vi "General Error Handler CORE.vi"(0 "[error code] (0)":i32 format="%0.0f", 1 "[user-defined codes]":i32[](array[numeric]), 2 "[user-defined descriptions]":string[](array[string]), 5 "[error source] (\" \")":string, 7 "String to Format (not a refnum)":refnum<vi>, 9 "type of dialog (OK msg:1)":T2=enum."OK message", 11 "error in (no error)":errorcluster, 12 "[exception action] (none:0)":i32(ring) items=["no exception", "cancel error on match", "set error on match"], 13 "[exception code]":i32 format="%0.0f", 14 "[exception source]":string) -> (3 "stop event propagated":bool, 4 "error?":bool, 6 "code out":i32 format="%0.0f", 8 "source out":string, 10 "message":string=" INSTRUCTIONS:\r\rNormal Use:  When using subVIs that incorporate the error in/error out (or error I/O) structure, place this handler where you want to inform the user of an error, typically at the end of the I/O data path, as the last action of the program.  If the error in error? is ERROR, the handler creates a message describing the error and its source.  If the type of dialog = 1 (default), the message is displayed to the user, who can only acknowledge it.  If the type = 2, the user can acknowledge the message or abort execution; aborting a program with active I/O is not recommended.  If the type = 0, no message is displayed; this is used to process the error programmatically, and the error out cluster elements are wired to individual terminals for that reason.  \r\rOther Use:\n\r\nlocal testing.  To test the error code of a subVI or function that does not have the error I/O structure, you can wire its error code and a source string to the local error code and error source inputs.  If error in error? indicates no error and error code is not equal to 0, the local code and source are substituted for the error in values, and error? is set TRUE (ERROR).", 15 "error out":errorcluster)   [LabVIEW 2011]
doc: "Indicates whether an error occurred. If an error occurred, this VI returns a description of the error and optionally displays a dialog box."
uses:
  DialogTypeEnum.ctl
  whitespace.ctl
panel:
  in  "prompts":T1={"Error %d occurred at %s"="Error %d occurred at %s", "Warning %d occurred at %s"="Warning %d occurred at %s", "Possible reasons: %s"="<b>Possible reason(s):</b>\\n%s", "Error not listed"="This error code is undefined. No one has provided a description for this code, or you might have wired a number that is not an error code to the error code input.", "GetCommError x%lx"="Windows GetCommError:  The hex value of this code is <B>x%04lx</B>.\n\nInterpret it bit-wise as follows:\n<B>x4000</B>: serial port VI error\n<B>x0001</B>: receiving queue overflowed or character was received after end-of-file character\n<B>x0002</B>: character was lost by overwrite\n<B>x0004</B>: parity error\n<B>x0008</B>: framing error\n<B>x0010</B>: break condition\n<B>x0020</B>: CTS timeout\n<B>x0040</B>: DSR timeout\n<B>x0080</B>: RLSD timeout\n<B>x0100</B>: transmission queue was full when new character arrived\n<B>x0200</B>: parallel device timeout\n<B>x0400</B>: parallel device I/O error\n<B>x0800</B>: parallel device not selected\n<B>x1000</B>: parallel device out of paper\n<B>x8000</B>: requested mode is  not supported or the idComDev parameter is invalid.", "Continue"="Continue", "Stop"="Stop", "an unidentified location"="an unidentified location", "No Error"="No Error", "Help"="Why not found?"}
  # "reinitialize to default to display instructions"
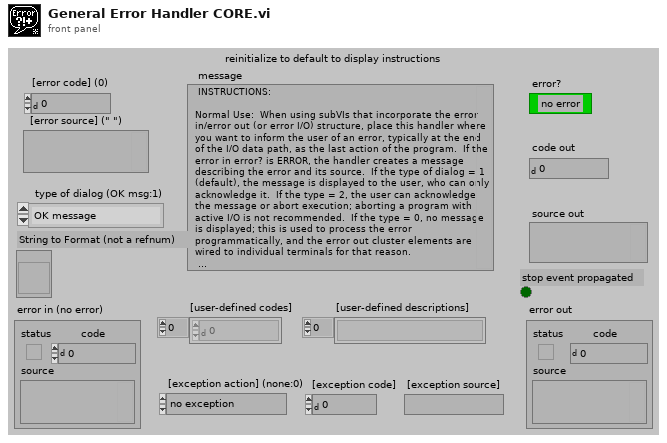
[diagram p1: front panel]
types:
  T1 = cluster{"Error %d occurred at %s":string, "Warning %d occurred at %s":string, "Possible reasons: %s":string, "Error not listed":string, "GetCommError x%lx":string, "Continue":string, "Stop":string, "an unidentified location":string, "No Error":string, "Help":string}
  T2 = typedef "DialogTypeEnum.ctl" = enum16{"no dialog", "OK message", "continue or stop message", "auto error handling dialog", "OK message + warnings", "continue/stop + warnings"}
  T3 = typedef "TagReturnType.ctl" = enum16{"No Tag", "<err>", "<append>"}
  T4 = typedef "whitespace.ctl" = u16
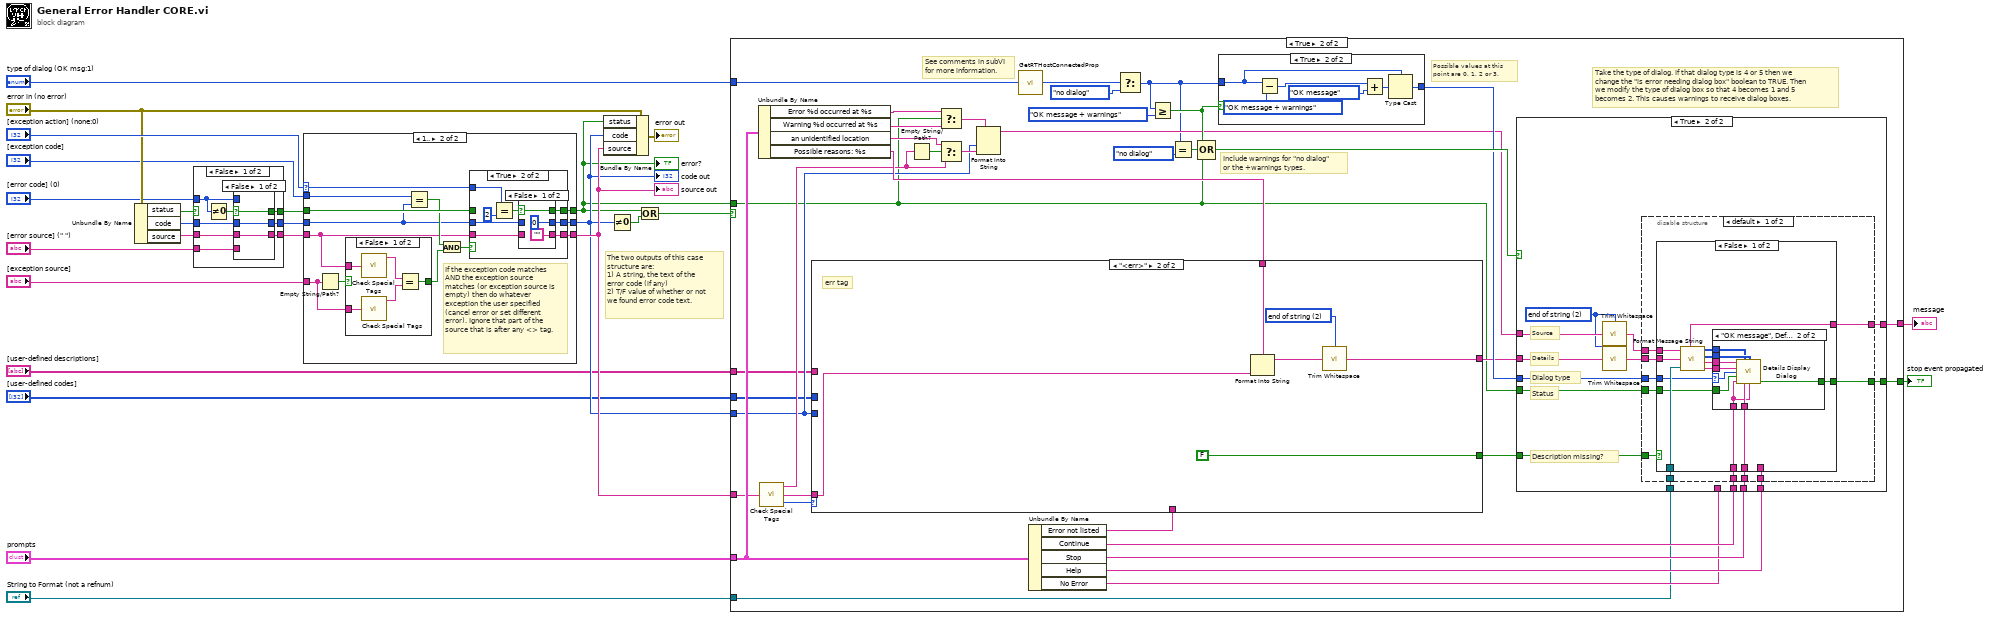
[diagram p0: block diagram]
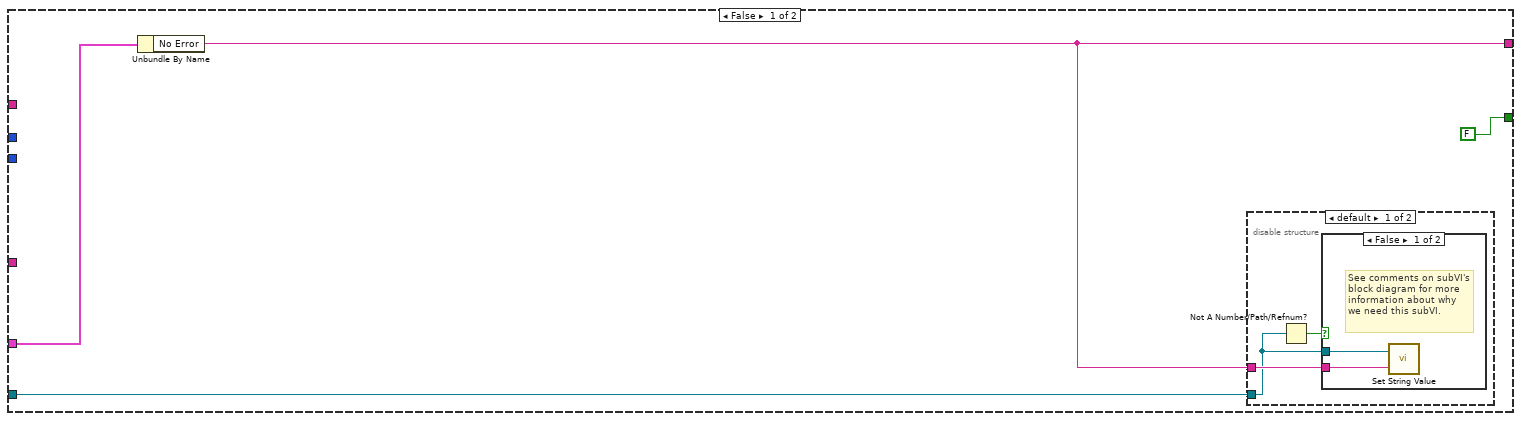
[diagram p8: hidden frame]
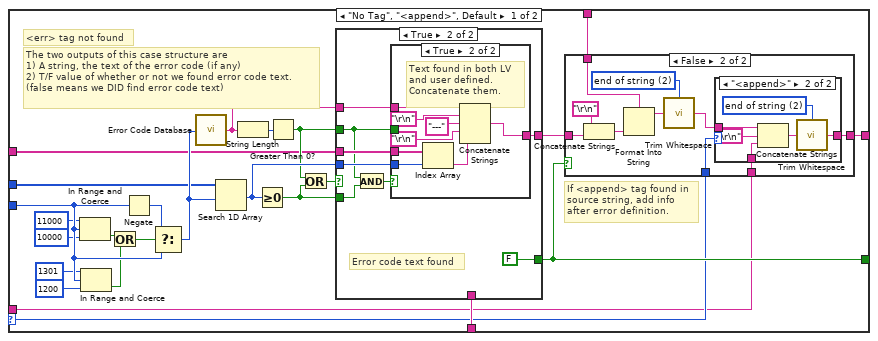
[diagram p12: hidden frame]
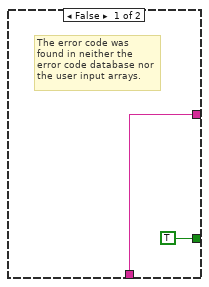
[diagram p15: hidden frame]
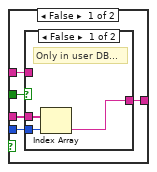
[diagram p16: hidden frame]
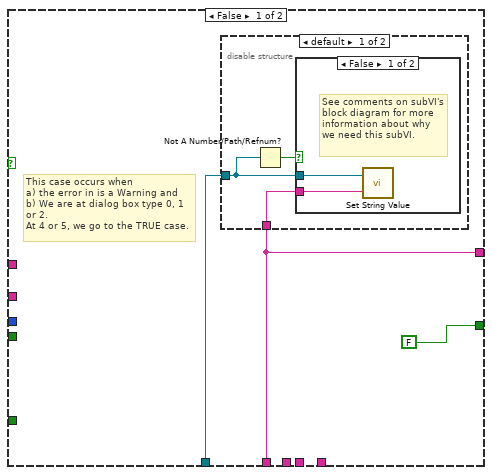
[diagram p18: hidden frame]
diagram:
  # "The two outputs of this case structure are:\n1) A string, the text of the error code (if any)\n2) T/F value of whether or not we found error code text."
  n1 = Unbundle By Name("error in (no error)") -> ("status"=w6:bool, "code"=w20:i32, "source"=w24:string)
  n2 = case shown="False" w6 {
    selector: w6 -> [_ w42]
    tunnel: [w31 w41] -> w22
    tunnel: [w32 w42] -> w21
    tunnel: w20 -> [w28 w41]
    tunnel: [w30 w40] -> w23
    tunnel: w24 -> [w29 w40]
    tunnel: "[error code] (0)" -> [w27 _]
    tunnel: "[error source] (\" \")" -> [w26 _]
    frame False {
      n3 = Not Equal To 0?(x=w27) -> (x != 0?=w33:bool)
      n4 = case shown="False" w33 {
        selector: w33 -> [w36 w39]
        tunnel: [w36 w39] -> w32
        tunnel: w27 -> [_ w38]
        tunnel: [w34 w38] -> w31
        tunnel: w26 -> [_ w37]
        tunnel: [w35 w37] -> w30
        tunnel: w29 -> [w35 _]
        tunnel: w28 -> [w34 _]
        frame False {
        }
        frame True {
        }
      }
    }
    frame True {
    }
  }
  n5 = case shown="1.." "[exception action] (none:0)" {
    selector: "[exception action] (none:0)" -> [_ w50]
    tunnel: [w45 w58] -> w2
    tunnel: w21 -> [w45 w56]
    tunnel: [w44 w57] -> w7
    tunnel: w22 -> [w44 w54]
    tunnel: [w43 w52] -> w17
    tunnel: w23 -> [w43 w48]
    tunnel: "[exception code]" -> [_ w51]
    tunnel: "[exception source]" -> [_ w47]
    frame ..0 {
    }
    frame 1.. {
      # "If the exception code matches AND the exception source matches (or exception source is empty) then do whatever exception the user specified (cancel error or set different error). Ignore that part of the source that is after any <> tag."
      n6 = Empty String/Path?(string/path=w47) -> (empty?=w49:bool)
      n7 = case shown="False" w49 {
        selector: w49 -> [_ w64]
        tunnel: w48 -> [w63 _]
        tunnel: w47 -> [w62 _]
        tunnel: [w61 w64] -> w46
        frame False {
          n8 = call "Check Special Tags.vi"("source"=w63) -> ("Before Tag (source)"=w60:string)  [unwired: 2 out]
          n9 = call "Check Special Tags.vi"("source"=w62) -> ("Before Tag (source)"=w59:string)  [unwired: 2 out]
          n10 = Equal?(x=w60, y=w59) -> (x = y?=w61:bool)
        }
        frame True {
          # "Empty string always matches."
        }
      }
      n11 = Equal?(x=w51, y=w54) -> (x = y?=w55:bool)
      n12 = And(x=w55, y=w46) -> (x .and. y?=w53:bool)
      n13 = case shown="True" w53 {
        tunnel: [w67 w68] -> w58
        tunnel: [w66 w72] -> w57
        tunnel: w56 -> [w67 _]
        tunnel: w54 -> [w66 w71]
        tunnel: w50 -> [_ w75]
        tunnel: [w65 w70] -> w52
        tunnel: w48 -> [w65 w69]
        frame False {
        }
        frame True {
          n14 = Equal?(x=w75, y=2) -> (x = y?=w73:bool)
          n15 = case shown="False" w73 {
            selector: w73 -> [w78 w81]
            tunnel: [0 w80] -> w72
            tunnel: w71 -> [_ w80]
            tunnel: ["" ("Empty String Constant") w79] -> w70
            tunnel: w69 -> [_ w79]
            tunnel: [w78 w81] -> w68
            frame False {
            }
            frame True {
            }
          }
        }
      }
    }
  }
  "source out" <- w17
  "error?" <- w2
  "code out" <- w7
  n16 = Bundle By Name(cluster="error in (no error)", "status"=w2, "code"=w7, "source"=w17) -> (→"error out":errorcluster)
  n17 = Not Equal To 0?(x=w7) -> (x != 0?=w1:bool)
  n18 = Or(x=w2, y=w1) -> (x .or. y?=w18:bool)
  n19 = case shown="True" w18 {
    tunnel: [w83 w109] -> w25
    tunnel: w2 -> [_ w91]
    tunnel: w17 -> [_ w99]
    tunnel: "prompts" -> [w85 w118]
    tunnel: [FALSE ("Stop 2") w112] -> w13
    tunnel: "String to Format (not a refnum)" -> [w82 w105]
    tunnel: w7 -> [_ w97]
    tunnel: "[user-defined descriptions]" -> [_ w95]
    tunnel: "[user-defined codes]" -> [_ w94]
    tunnel: "type of dialog (OK msg:1)" -> [_ w93]
    frame False {
      n20 = Unbundle By Name(w85) -> ("No Error"=w83:string)
      n21 = disable-structure shown="default" {
        disable-tunnel: w83 -> [w88 _]
        disable-tunnel: w82 -> [w87 _]
        frame condition #0 (active) {
          n22 = Not A Number/Path/Refnum?(number/path/refnum=w87) -> (NaN/Path/Refnum?=w86:bool)
          n23 = case shown="False" w86 {
            tunnel: w88 -> [w90 _]
            tunnel: w87 -> [w89 _]
            frame False {
              # "See comments on subVI's block diagram for more information about why we need this subVI."
              n24 = call "Set String Value.vi"("No Error"=w90, "String to Format (not a refnum)"=w89) -> ()
            }
            frame True {
            }
          }
        }
        frame condition #1 {
          # "Do nothing in RT case."
        }
      }
    }
    frame True {
      # "See comments in subVI for more information."
      # "Include warnings for \"no dialog\" or the +warnings types."
      # "Possible values at this point are 0, 1, 2 or 3."
      # "Take the type of dialog. If that dialog type is 4 or 5 then we change the \"is error needing dialog box\" boolean to TRUE. Then we modify the type of dialog box so that 4 becomes 1 and 5 becomes 2. This causes warnings to receive dialog boxes."
      n25 = Unbundle By Name(w118) -> ("Error %d occurred at %s"=w96:string, "Warning %d occurred at %s"=w125:string, "an unidentified location"=w122:string, "Possible reasons: %s"=w111:string)
      n26 = call "Check Special Tags.vi"("source"=w99) -> ("Before Tag (source)"=w98:string, "After Tag (special data)"=w126:string, "Tag Found?"=w113:T3)
      n27 = Empty String/Path?(string/path=w98) -> (empty?=w127:bool)
      n28 = Select(t=w96, s=w91, f=w125) -> (s? t:f=w124:string)
      n29 = Select(t=w122, s=w127, f=w98) -> (s? t:f=w123:string)
      n30 = Format Into String(format string=w124, w97, w123) -> (resulting string=w107:string)  [unwired: 2 in, 1 out]
      n31 = call "GetRTHostConnectedProp.vi"() -> ("App.RTHostConnected"=w92:bool)
      n32 = Unbundle By Name(w118) -> ("Error not listed"=w121:string, "Continue"=w120:string, "Stop"=w119:string, "Help"=w116:string, "No Error"=w106:string)
      n33 = case shown="\"<err>\"" w113 {
        selector: w113 -> [w140 _]
        tunnel: [w138 w208] -> w108
        tunnel: w97 -> [w159 _]
        tunnel: w126 -> [w139 w207]
        tunnel: w121 -> [w158 _]
        tunnel: [w141 FALSE] -> w117
        tunnel: w111 -> [w143 w206]
        tunnel: w95 -> [w136 _]
        tunnel: w94 -> [w135 _]
        frame "No Tag", "<append>", Default {
          # "If <append> tag found in source string, add info after error definition."
          # "<err> tag not found"
          # "The two outputs of this case structure are\n1) A string, the text of the error code (if any)\n2) T/F value of whether or not we found error code text.\n(false means we DID find error code text)"
          n34 = In Range and Coerce(upper limit=11000, x=w159, lower limit=10000) -> (In Range?=w151:bool)  [unwired: 1 out]
          n35 = In Range and Coerce(upper limit=1301, x=w159, lower limit=1200) -> (In Range?=w152:bool)  [unwired: 1 out]
          n36 = Or(x=w151, y=w152) -> (x .or. y?=w150:bool)
          n37 = Negate(x=w159) -> (-x=w154:i32)
          n38 = Select(t=w154, s=w150, f=w159) -> (s? t:f=w137:i32)
          n39 = call "Error Code Database.vi"("Error Code"=w137) -> ("Error Text"=w144:string)
          n40 = Search 1D Array(1D array=w135, element=w137) -> (index of element=w157:i32)  [unwired: 1 out]
          n41 = String Length(string=w144) -> (length=w148:i32)
          n42 = Greater Or Equal To 0?(x=w157) -> (x >= 0?=w145:bool)
          n43 = Greater Than 0?(x=w148) -> (x > 0?=w146:bool)
          n44 = Or(x=w146, y=w145) -> (x .or. y?=w147:bool)
          n45 = case shown="True" w147 {
            tunnel: w157 -> [_ w183]
            tunnel: [w179 w181] -> w142
            tunnel: w158 -> [w179 _]
            tunnel: [TRUE FALSE] -> w141
            tunnel: w146 -> [_ w180]
            tunnel: w145 -> [_ w185]
            tunnel: w136 -> [_ w184]
            tunnel: w144 -> [_ w182]
            frame False {
              # "The error code was found in neither the error code database nor the user input arrays."
            }
            frame True {
              # "Error code text found"
              n46 = And(x=w180, y=w185) -> (x .and. y?=w186:bool)
              n47 = case shown="True" w186 {
                tunnel: w184 -> [w189 w204]
                tunnel: w183 -> [w188 w203]
                tunnel: w182 -> [w190 w197]
                tunnel: [w191 w201] -> w181
                tunnel: w180 -> [w192 _]
                frame False {
                  n48 = case shown="False" w192 {
                    tunnel: [w193 w196] -> w191
                    tunnel: w190 -> [_ w196]
                    tunnel: w189 -> [w195 _]
                    tunnel: w188 -> [w194 _]
                    frame False {
                      # "Only in user DB..."
                      n49 = Index Array(array=w195, index=w194) -> (element=w193:string)
                    }
                    frame True {
                      # "Only in LV DB..."
                    }
                  }
                }
                frame True {
                  # "Text found in both LV\nand user defined. \nConcatenate them."
                  n50 = Index Array(array=w204, index=w203) -> (element=w202:string)
                  n51 = Concatenate Strings(w197, "\r\n" ("End of Line Constant"), "---" ("string"), "\r\n" ("End of Line Constant"), w202) -> (w201:string)
                }
              }
            }
          }
          n52 = case shown="False" w141 {
            tunnel: w143 -> [_ w170]
            tunnel: [w160 w162] -> w138
            tunnel: w142 -> [w160 w167]
            tunnel: w140 -> [_ w164]
            tunnel: w139 -> [_ w163]
            frame True {
              # "no explanation given for error."
            }
            frame False {
              w161 = T4 2 items=["both", "start of string", "end of string"] ("location (both)")
              n53 = Concatenate Strings("\r\n" ("End of Line Constant"), w167) -> (w168:string)
              n54 = Format Into String(format string=w170, w168) -> (resulting string=w169:string)  [unwired: 2 in, 1 out]
              n55 = call "Trim Whitespace.vi"("string"=w169, "location (both)"=w161) -> ("trimmed string"=w165:string)
              n56 = case shown="\"<append>\"" w164 {
                tunnel: w165 -> [w171 w176]
                tunnel: [w171 w173] -> w162
                tunnel: w163 -> [_ w175]
                frame "No Tag", Default {
                }
                frame "<append>" {
                  w172 = T4 2 items=["both", "start of string", "end of string"] ("location (both)")
                  n57 = Concatenate Strings(w176, "\r\n" ("End of Line Constant"), w175) -> (w174:string)
                  n58 = call "Trim Whitespace.vi"("string"=w174, "location (both)"=w172) -> ("trimmed string"=w173:string)
                }
              }
            }
          }
        }
        frame "<err>" {
          w205 = T4 2 items=["both", "start of string", "end of string"] ("location (both)")
          # "err tag"
          n59 = Format Into String(format string=w206, w207) -> (resulting string=w209:string)  [unwired: 2 in, 1 out]
          n60 = call "Trim Whitespace.vi"("string"=w209, "location (both)"=w205) -> ("trimmed string"=w208:string)
        }
      }
      n61 = Select(t=w93, s=w92, f=DialogTypeEnum."no dialog" ("type of dialog (OK msg:1)")) -> (s? t:f=w100:T2)
      n62 = Greater Or Equal?(x=w100, y=DialogTypeEnum."OK message + warnings" ("type of dialog (OK msg:1)")) -> (x >= y?=w114:bool)
      n63 = Equal?(x=w100, y=DialogTypeEnum."no dialog" ("type of dialog (OK msg:1)")) -> (x = y?=w104:bool)
      n64 = Compound Arithmetic op=OR(w114, w104, w91) -> (w115:bool)
      n65 = case shown="True" w114 {
        tunnel: w100 -> [w128 w129]
        tunnel: [w128 w131] -> w110
        frame False {
        }
        frame True {
          n66 = Subtract(x=w129, y=DialogTypeEnum."OK message + warnings" ("type of dialog (OK msg:1)")) -> (x-y=w134:u16)
          n67 = Add(x=w134, y=DialogTypeEnum."OK message" ("type of dialog (OK msg:1)")) -> (x+y=w130:u16)
          n68 = Type Cast(type=w129, x=w130) -> (*(type *) &x=w131:T2)
        }
      }
      n69 = case shown="True" w115 {
        tunnel: w110 -> [_ w232]
        tunnel: w120 -> [_ w231]
        tunnel: w119 -> [_ w230]
        tunnel: w117 -> [_ w219]
        tunnel: w116 -> [_ w229]
        tunnel: w107 -> [_ w222]
        tunnel: w108 -> [_ w223]
        tunnel: w91 -> [_ w228]
        tunnel: [FALSE ("Stop 2") w227] -> w112
        tunnel: [w211 w226] -> w109
        tunnel: w106 -> [w211 _]
        tunnel: w105 -> [w212 w225]
        frame False {
          # "This case occurs when\na) the error in is a Warning and\nb) We are at dialog box type 0, 1 or 2.\nAt 4 or 5, we go to the TRUE case."
          n70 = disable-structure shown="default" {
            disable-tunnel: w212 -> [w216 _]
            disable-tunnel: w211 -> [w214 _]
            frame condition #0 (active) {
              n71 = Not A Number/Path/Refnum?(number/path/refnum=w216) -> (NaN/Path/Refnum?=w215:bool)
              n72 = case shown="False" w215 {
                tunnel: w214 -> [w218 _]
                tunnel: w216 -> [w217 _]
                frame False {
                  # "See comments on subVI's block diagram for more information about why we need this subVI."
                  n73 = call "Set String Value.vi"("No Error"=w218, "String to Format (not a refnum)"=w217) -> ()
                }
                frame True {
                }
              }
            }
            frame condition #1 {
              # "Do nothing in RT case."
            }
          }
        }
        frame True {
          w220 = T4 2 items=["both", "start of string", "end of string"] ("location (both)")
          # "Description missing?"
          # "Dialog type"
          # "Status"
          # "Details"
          # "Source"
          n74 = call "Trim Whitespace.vi"("string"=w222, "location (both)"=w220) -> ("trimmed string"=w221:string)
          n75 = call "Trim Whitespace.vi"("string"=w223, "location (both)"=w220) -> ("trimmed string"=w224:string)
          n76 = disable-structure "Conditional Disable Structure" shown="default" {
            disable-tunnel: w232 -> [w243 w287]
            disable-tunnel: w231 -> [w242 w286]
            disable-tunnel: w230 -> [w241 w285]
            disable-tunnel: w229 -> [w240 _]
            disable-tunnel: w228 -> [w239 _]
            disable-tunnel: [w238 w284] -> w227
            disable-tunnel: [w237 w283] -> w226
            disable-tunnel: w225 -> [w236 w282]
            disable-tunnel: w224 -> [w235 w281]
            disable-tunnel: w221 -> [w234 w280]
            disable-tunnel: w219 -> [w233 _]
            frame condition #0 (active) {
              n77 = case shown="False" w233 {
                tunnel: w235 -> [w255 w271]
                tunnel: w240 -> [_ w277]
                tunnel: w242 -> [w251 w275]
                tunnel: w241 -> [w250 w274]
                tunnel: w243 -> [w253 w276]
                tunnel: [w252 w273] -> w238
                tunnel: w234 -> [w256 w272]
                tunnel: w239 -> [w249 _]
                tunnel: [w244 w269] -> w237
                tunnel: w236 -> [w254 w267]
                frame False {
                  n78 = call "Format Message String.vi"("Source"=w256, "Details"=w255, "String to Format (not a refnum)"=w254) -> ("message"=w244:string, "Bold Start"=w248:i32[], "Bold Length"=w247:i32[], "Source Out"=w246:string, "Details Out"=w245:string)  [unwired: 1 out]
                  n79 = case shown="\"OK message\", Default" w253 {
                    selector: w253 -> [_ w263]
                    tunnel: [FALSE ("stop event propagated") w266] -> w252
                    tunnel: w251 -> [_ w264]
                    tunnel: w250 -> [_ w265]
                    tunnel: w249 -> [_ w262]
                    tunnel: w248 -> [_ w258]
                    tunnel: w247 -> [_ w261]
                    tunnel: w246 -> [_ w260]
                    tunnel: w245 -> [_ w259]
                    frame "no dialog" {
                    }
                    frame "OK message", Default {
                      n80 = call "Details Display Dialog.vi"("Source"=w260, "Start"=w258, "Length"=w261, "Details"=w259, "dialog type"=w263, "Error or Warning"=w262, "contname"=w264, "stopname"=w265, "okname"=w264) -> ("stop event propagated"=w266:bool)  [unwired: 6 out]
                    }
                  }
                }
                frame True {
                  w270 = "\r\n" ("End of Line Constant")
                  n81 = Concatenate Strings(w272, w270, w270, w271) -> (w269:string)
                  n82 = Not A Number/Path/Refnum?(number/path/refnum=w267) -> (NaN/Path/Refnum?=w268:bool)
                  n83 = call "Not Found Dialog.vi"("Help"=w277, "Message"=w269, "Stop"=w274, "Continue"=w275, "type of dialog (OK msg:1)"=w276) -> ("stop event propagated"=w273:bool)  [unwired: 1 in]
                  n84 = case shown="False" w268 {
                    tunnel: w267 -> [w279 _]
                    tunnel: w269 -> [w278 _]
                    frame False {
                      n85 = call "Set String Value.vi"("No Error"=w278, "String to Format (not a refnum)"=w279) -> ()
                    }
                    frame True {
                    }
                  }
                }
              }
            }
            frame condition #1 {
              n86 = call "Format Message String.vi"("Source"=w280, "Details"=w281, "String to Format (not a refnum)"=w282) -> ("message"=w283:string)  [unwired: 1 in, 4 out]
              n87 = case shown="\"continue or stop message\", \"continue/stop + warnings\"" w287 {
                tunnel: [FALSE ("stop event propagated") FALSE ("stop event propagated") FALSE ("stop event propagated") w298] -> w284
                tunnel: w283 -> [_ w290 w297 w302]
                tunnel: w286 -> [_ w289 w296 w301]
                tunnel: w285 -> [_ _ w295 w300]
                frame "no dialog" {
                }
                frame "OK message", "OK message + warnings", Default {
                  n88 = One Button Dialog(message=w290, button name ("OK")=w289) -> ()  [unwired: 1 out]
                }
                frame "continue or stop message", "continue/stop + warnings" {
                  n89 = Two Button Dialog(message=w297, 1:w295, 2:w296) -> (T button?=w293:bool)
                  n90 = Not(x=w293) -> (.not. x?=w292:bool)
                  n91 = Stop(stop? (T)=w292) -> ()
                }
                frame "auto error handling dialog" {
                  n92 = Two Button Dialog(message=w302, 1:w300, 2:w301) -> (T button?=w299:bool)
                  n93 = Not(x=w299) -> (.not. x?=w298:bool)
                }
              }
            }
          }
        }
      }
    }
  }
  "message" <- w25
  "stop event propagated" <- w13
